vi "GetPigeonIMU.vi"(4 "Pose Mode":T1(ring)) -> (5 "Yaw (deg)":dbl format="%#_13g", 6 "Yaw Rate (deg/s)":dbl format="%#_13g", 7 "Pitch (deg)":dbl format="%#_13g")   [LabVIEW 2023]
doc: "This VI reads the Pigeon IMU yaw and yaw rate values. It also handles error detection and orientation resets and supports simulation of the IMU to facilitate auto testing."
uses:
  GlobalDriverStationData.vi
  GlobalDrivebase.vi
  GlobalPoseAndTargeting.vi
  <vilib>/Rock Robotics/WPI/ThirdParty/Phoenix-LabVIEW/Pigeon IMU/CTRE_PigeonIMU_GetRawGyro.vi
  <vilib>/Rock Robotics/WPI/ThirdParty/Phoenix-LabVIEW/Pigeon IMU/CTRE_PigeonIMU_GetYPR.vi
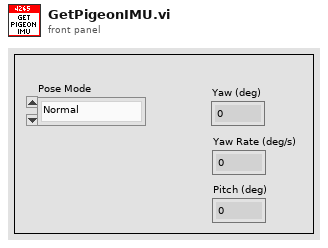
[diagram p1: front panel]
types:
  T1 = enum16{"Normal", "Auto Set", "Reset IMU", "Manual Push", "Init"}
  T2 = typedef "CTRE_PigeonIMU_DeviceRef.ctl" = cluster{"DeviceStatus":errorcluster, "Device Number":u8, "Type":T3, "Device ID":u32, "Handle":u64, "UsageFrame":u32, "Library Path":path}
  T3 = typedef "CTRE_PigeonIMU_ConnectionType.ctl" = u32
  T4 = typedef "WPI_DriverStationAllianceInfo.ctl" = enum16{"Red", "Blue", "Invalid"}
  T5 = cluster{"X":dbl, "Y":dbl, "Z":dbl, "Magnitude":dbl}
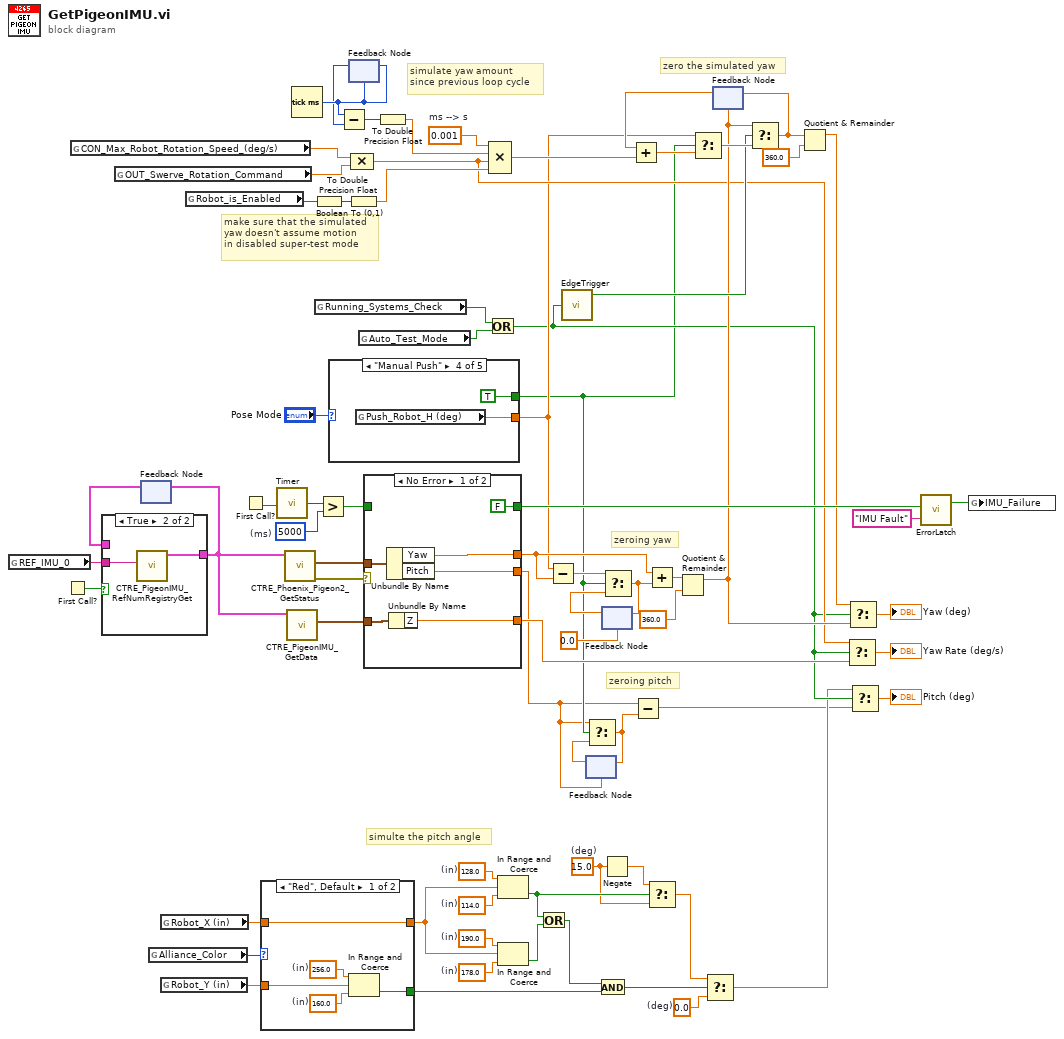
[diagram p0: block diagram]
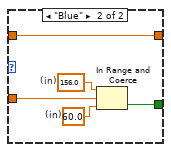
[diagram p2: hidden frame]
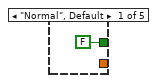
[diagram p3: hidden frame]
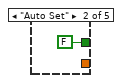
[diagram p4: hidden frame]
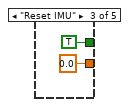
[diagram p5: hidden frame]
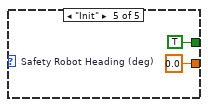
[diagram p6: hidden frame]
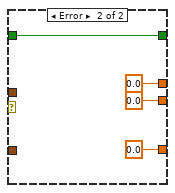
[diagram p7: hidden frame]
diagram:
  w7 = 15.0  # (deg)
  w10 = 0.0  # (deg)
  w21 = 178.0  # (in)
  w20 = 190.0  # (in)
  w19 = 114.0  # (in)
  w18 = 128.0  # (in)
  w38 = 0.001  # ms --> s
  w58 = u32 5000  # (ms)
  # "zeroing pitch"
  # "simulte the pitch angle"
  # "zero the simulated yaw"
  # "zeroing yaw"
  # "make sure that the simulated\nyaw doesn't assume motion\nin disabled super-test mode"
  # "simulate yaw amount\nsince previous loop cycle"
  n1 = global read "GlobalDrivebase.vi" "REF_IMU_0"() -> (w29:string)
  n2 = First Call?() -> (First Call?: T/F=w63:bool)
  n3 = global read "GlobalDrivebase.vi" "CON_Max_Robot_Rotation_Speed_(deg/s)"() -> (w28:dbl)
  n4 = global read "GlobalDrivebase.vi" "OUT_Swerve_Rotation_Command"() -> (w27:dbl)
  n5 = feedback #1() -> (w73:T2)  [unwired: 1 in]
  n6 = case shown="True" w63 {
    tunnel: [w74 w76] -> w55
    tunnel: w73 -> [w74 _]
    tunnel: w29 -> [_ w75]
    frame False {
    }
    frame True {
      n7 = call <vilib>:"CTRE_PigeonIMU_RefNumRegistryGet.vi"("refnum name"=w75) -> ("PigeonIMUDevRef"=w76:T2)  [unwired: 9 in, 1 out]
    }
  }
  n8 = feedback-in #1(w55) -> ()
  n9 = global read "GlobalDriverStationData.vi" "Alliance_Color"() -> (w23:T4)
  n10 = global read "GlobalPoseAndTargeting.vi" "Robot_X (in)"() -> (w17:dbl)
  n11 = global read "GlobalPoseAndTargeting.vi" "Robot_Y (in)"() -> (w22:dbl)
  n12 = global read "GlobalDriverStationData.vi" "Robot_is_Enabled"() -> (w26:bool)
  n13 = First Call?() -> (First Call?: T/F=w60:bool)
  n14 = case shown="\"Red\", Default" w23 {
    tunnel: w22 -> [w81 w86]
    tunnel: w17 -> [w78 w83]
    tunnel: [w78 w83] -> w16
    tunnel: [w77 w82] -> w14
    frame "Red", Default {
      w79 = 160.0  # (in)
      w80 = 256.0  # (in)
      n15 = In Range and Coerce(upper limit=w80, x=w81, lower limit=w79) -> (In Range?=w77:bool)  [unwired: 1 out]
    }
    frame "Blue" {
      w84 = 60.0  # (in)
      w85 = 156.0  # (in)
      n16 = In Range and Coerce(upper limit=w85, x=w86, lower limit=w84) -> (In Range?=w82:bool)  [unwired: 1 out]
    }
  }
  n17 = call "Timer.vi"("Reset Timer"=w60) -> ("Time (ms)"=w59:u32)
  n18 = call-poly <vilib>:"CTRE_Phoenix_Pigeon2_GetStatus.vi"("PigeonIMUDevRef"=w55) -> ("error out"=w62:errorcluster, "Yaw Pitch Roll"=w61:cluster{"Yaw":dbl, "Pitch":dbl, "Roll":dbl})  [unwired: 8 in, 1 out]
  n19 = call-poly <vilib>:"CTRE_PigeonIMU_GetData.vi"("PigeonIMUDevRef"=w55) -> ("Gyro DPS"=w54:T5)  [unwired: 8 in, 2 out]
  n20 = Tick Count (ms)() -> (millisecond timer value=w42:u32)
  n21 = Boolean To (0,1)(Boolean=w26) -> (0, 1=w45:i16)
  n22 = global read "GlobalDriverStationData.vi" "Running_Systems_Check"() -> (w52:bool)
  n23 = Greater?(x=w59, y=w58) -> (0:w57:bool)
  n24 = case shown="\"Manual Push\"" "Pose Mode" {
    tunnel: [_ _ 0.0 ("Push_Robot_H (deg)") w92 w93] -> w31
    tunnel: [FALSE FALSE TRUE TRUE TRUE] -> w4
    frame "Normal", Default {
    }
    frame "Auto Set" {
    }
    frame "Reset IMU" {
    }
    frame "Manual Push" {
      n25 = global read "GlobalPoseAndTargeting.vi" "Push_Robot_H (deg)"() -> (w92:dbl)
    }
    frame "Init" {
      w93 = 0.0  # Safety Robot Heading (deg)
    }
  }
  n26 = feedback #2(w42) -> (w41:u32)
  n27 = Subtract(x=w42, y=w41) -> (x-y=w40:u32)
  n28 = feedback-in #2(w42) -> ()
  n29 = To Double Precision Float(number=w45) -> (double precision float=w46:dbl)
  n30 = Compound Arithmetic op=MULTIPLY(w28, w27) -> (w32:dbl)
  n31 = global read "GlobalDriverStationData.vi" "Auto_Test_Mode"() -> (w53:bool)
  n32 = case shown="No Error" w62 {
    tunnel: [FALSE w102] -> w66
    tunnel: w61 -> [w99 _]
    tunnel: [w98 0.0 ("Yaw")] -> w64
    tunnel: w57 -> [_ w102]
    tunnel: [w97 0.0 ("X")] -> w50
    tunnel: w54 -> [w96 _]
    tunnel: [w95 0.0 ("Pitch")] -> w3
    frame No Error {
      n33 = Unbundle By Name(w99) -> ("Yaw"=w98:dbl, "Pitch"=w95:dbl)
      n34 = Unbundle By Name(w96) -> ("Z"=w97:dbl)
    }
    frame Error {
    }
  }
  n35 = To Double Precision Float(number=w40) -> (double precision float=w39:dbl)
  n36 = Or(x=w52, y=w53) -> (x .or. y?=w24:bool)
  n37 = Compound Arithmetic op=MULTIPLY(w38, w39, w32, w46) -> (w47:dbl)
  n38 = In Range and Coerce(upper limit=w18, x=w16, lower limit=w19) -> (In Range?=w12:bool)  [unwired: 1 out]
  n39 = In Range and Coerce(upper limit=w20, x=w16, lower limit=w21) -> (In Range?=w15:bool)  [unwired: 1 out]
  n40 = Or(x=w12, y=w15) -> (x .or. y?=w13:bool)
  n41 = Subtract(x=w31, y=w64) -> (x-y=w72:dbl)
  n42 = call "EdgeTrigger.vi"("Input Signal"=w24) -> ("Rising Edge Trigger"=w34:bool)  [unwired: 2 out]
  n43 = feedback #3(w3) -> (w6:dbl)
  n44 = Select(t=w3, s=w4, f=w6) -> (s? t:f=w5:dbl)
  n45 = feedback-in #3(w5) -> ()
  n46 = And(x=w13, y=w14) -> (x .and. y?=w11:bool)
  n47 = feedback #4(0.0) -> (w71:dbl)
  n48 = Negate(x=w7) -> (-x=w1:dbl)
  n49 = Select(t=w72, s=w4, f=w71) -> (s? t:f=w69:dbl)
  n50 = feedback-in #4(w69) -> ()
  n51 = Subtract(x=w3, y=w5) -> (x-y=w2:dbl)
  n52 = Add(x=w64, y=w69) -> (x+y=w67:dbl)
  n53 = Select(t=w1, s=w12, f=w7) -> (s? t:f=w9:dbl)
  n54 = Quotient & Remainder(x=w67, y=360.0) -> (x-y*floor(x/y)=w33:dbl)  [unwired: 1 out]
  n55 = Select(t=w9, s=w11, f=w10) -> (s? t:f=w8:dbl)
  n56 = feedback #5(w33) -> (w43:dbl)
  n57 = Add(x=w43, y=w47) -> (x+y=w37:dbl)
  n58 = Select(t=w31, s=w4, f=w37) -> (s? t:f=w36:dbl)
  n59 = Select(t=w33, s=w34, f=w36) -> (s? t:f=w35:dbl)
  n60 = feedback-in #5(w35) -> ()
  n61 = Quotient & Remainder(x=w35, y=360.0) -> (x-y*floor(x/y)=w48:dbl)  [unwired: 1 out]
  n62 = Select(t=w32, s=w24, f=w50) -> (s? t:f=→"Yaw Rate (deg/s)":dbl)
  n63 = Select(t=w48, s=w24, f=w33) -> (s? t:f=→"Yaw (deg)":dbl)
  n64 = Select(t=w8, s=w24, f=w2) -> (s? t:f=→"Pitch (deg)":dbl)
  n65 = call "ErrorLatch.vi"("Error Message"="IMU Fault", "Trigger"=w66) -> ("Latched"=w65:bool)  [unwired: 1 in]
  n66 = global write "GlobalPoseAndTargeting.vi" "IMU_Failure"(w65) -> ()
